vi "setDAC.vi"(8 "error in (no error)":errorcluster, 9 "DAC Value":u16, 10 "ILC in":refnum<class "ILC.lvclass">, 11 "IILCDAC in":refnum<class "IILCDAC.lvclass">) -> (0 "error out":errorcluster, 2 "ILC out":refnum<class "ILC.lvclass">, 3 "IILCDAC out":refnum<class "IILCDAC.lvclass">)   [LabVIEW 2015, in "IILCDAC.lvclass"]
uses:
  IILCDAC.lvclass
  <userlib>/Common/ILC/ILC/ILC.lvclass
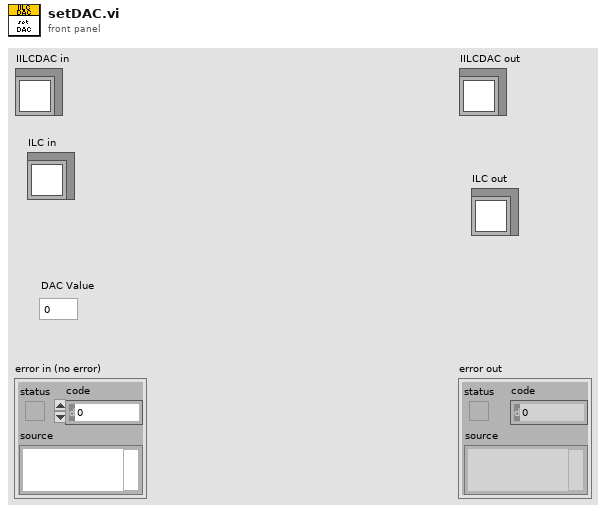
[diagram p1: front panel]
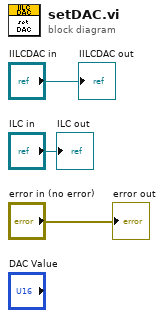
[diagram p0: block diagram]
diagram:
  "error out" <- "error in (no error)"
  "IILCDAC out" <- "IILCDAC in"
  "ILC out" <- "ILC in"
